vi "WriteSnapshot.vi"(0 "Buffers in":T1={"Channels"=[], "PosttriggerBuffer"=refnum, "PretriggerBuffer"=refnum, "BlockSizePerChannel"=0, " logging semaphore"=refnum, "Log refnum"=refnum, "snapshotBuffer"=refnum, "logDirectory"=path "", "logPrefix"="", "decimation factor"=1, "max files"=0, "SampleRate"=0.0}, 5 "Snapshot":sgl[](array[numeric]), 11 "error in (no error)":errorcluster) -> (4 "Buffers out":T1={"Channels"=[], "PosttriggerBuffer"=refnum, "PretriggerBuffer"=refnum, "BlockSizePerChannel"=0, " logging semaphore"=refnum, "Log refnum"=refnum, "snapshotBuffer"=refnum, "logDirectory"=path "", "logPrefix"="", "decimation factor"=1, "max files"=0, "SampleRate"=0.0}, 15 "error out":errorcluster)   [LabVIEW 2017, in "BufferLogging.lvlib"]
uses:
  BufferLogging.lvlib
  Buffers.ctl
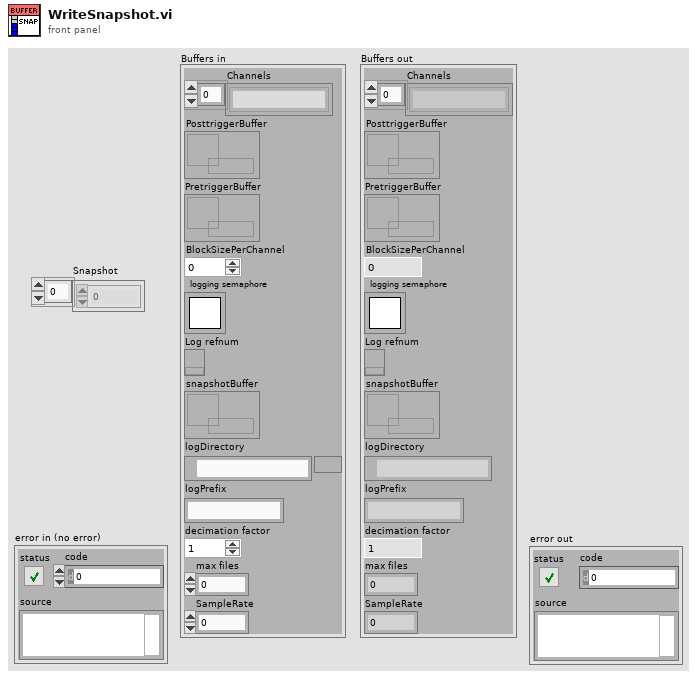
[diagram p1: front panel]
types:
  T1 = typedef "BufferLogging.lvlib/Buffers.ctl" = cluster{"Channels":string[], "PosttriggerBuffer":refnum<queue>, "PretriggerBuffer":refnum<queue>, "BlockSizePerChannel":i32, " logging semaphore":T2, "Log refnum":refnum<k34>, "snapshotBuffer":refnum<data-value>, "logDirectory":path, "logPrefix":string, "decimation factor":i32, "max files":i32, "SampleRate":dbl}
  T2 = typedef "Semaphore RefNum" = refnum<k1>
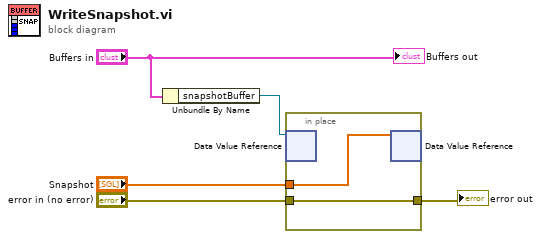
[diagram p0: block diagram]
diagram:
  n1 = Unbundle By Name("Buffers in") -> ("snapshotBuffer"=w4:refnum<data-value>)
  n2 = in-place {
    in-place-border: "Snapshot" -> [w7]
    in-place-border: "error in (no error)" -> [w6]
    in-place-border: [w6] -> w1
    n3 = in-place-dvr #1(w4) -> ()  [unwired: 2 out]
    n4 = in-place-dvr #1(w7) -> ()  [unwired: 2 out]
  }
  "error out" <- w1
  "Buffers out" <- "Buffers in"
